vi "Constants.vi"() -> ()   [LabVIEW 2020, in "AFPP Shared.lvlib"]
uses:
  AFPP Shared.lvlib
panel:
  in  "Actors":string="AF.Actors"
  in  "Actor Paths":string="AF.ActorPaths"
  in  "PPL Tag":string="AF.PPL"
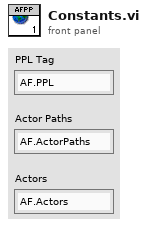
[diagram p1: front panel]
diagram:
